vi "PlatManipbyVoltage.vi"() -> ()   [LabVIEW 2015]
uses:
  <vilib>/picture/3D Picture Control/Object/Create Object (name).vi
  <vilib>/picture/3D Picture Control/NI_3D Picture Control.lvlib
panel:
  in  "Length Y":sgl=1.0
  in  "Length X":sgl=1.0
  in  "Length Z":sgl=1.0
  in  "Tamaño de la platina":cluster{"X":sgl, "Y":sgl, "Z":sgl}={"X"=1.457233, "Y"=1.0, "Z"=1.0} {"X" scale=0.0..5.0; "Y" scale=0.0..5.0; "Z" scale=0.0..5.0}
  out "Platina":refnum<vi>(3d-picture)
  out "data":dynamicdata(graph) caption="Voltaje"
  in  "stop":bool
  # "Manipulacion de una platina virtual"
  # "Serrano Bermúdez Luis Esteban\nFecha de Entrega 13/04/2019"
  # "Descripcion:"
  # "Esta aplicacion simula una platina con un objeto 3D de una caja la cual\nse puede mover con el uso de potenciometros conectados a la tarjeta\nDAQ a partir de la medicion de voltaje a la salida de la terminal central\ndel potenciometro.\nLas gráficas del lado derecho muestra la variación del voltaje y la\ngráfica del lado derecho simula una platina que se moverá\ndependiendo del potenciometro."
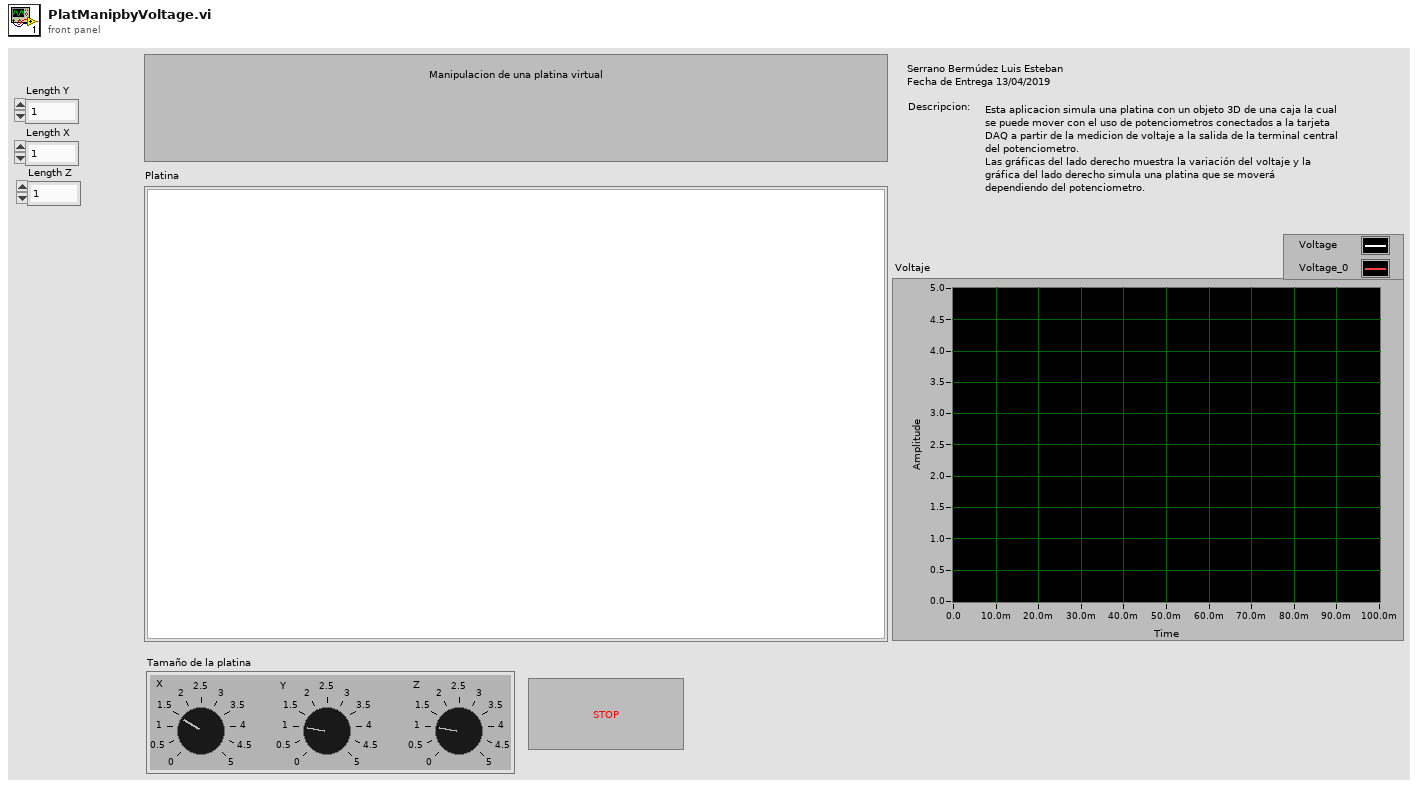
[diagram p1: front panel]
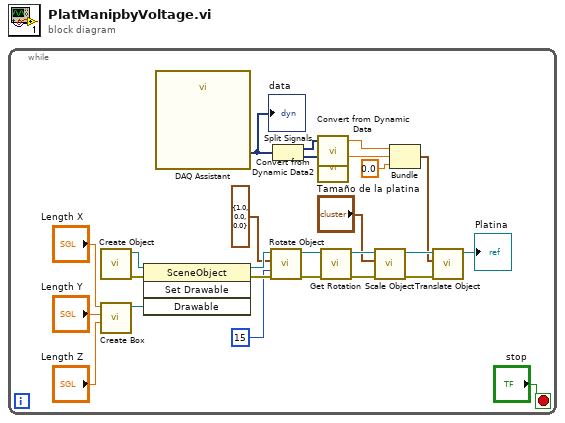
[diagram p0: block diagram]
diagram:
  n1 = while {
    stop <- "stop" stop-if-true
    n2 = call-poly <vilib>:"Create Object.vi"() -> ("error out"=w24:errorcluster, "Scene:New Object"=w25:refnum<vi>)  [unwired: 10 in]
    n3 = call <vilib>:"Create Box.vi"("Length Z"="Length Z", "Length Y"="Length Y", "Length X"="Length X") -> ("New Box Refnum"=w23:refnum<vi>)  [unwired: 7 in, 1 out]
    n4 = invoke class="SceneObject" method="Set Drawable"(reference=w25, error in=w24, "Drawable"=w23) -> (reference out=w19:refnum<vi>, error out=w18:errorcluster)  [unwired: 1 in, 2 out]
    n5 = call "DAQ Assistant"() -> ("data"=w5:dynamicdata)  [unwired: 17 in, 2 out]
    "data" <- w5
    n6 = call <vilib>:"Rotate Object.vi"("error in (no error)"=w18, "Angle"=15, "Axis"=cluster{"X":sgl, "Y":sgl, "Z":sgl} {"X"=1.0, "Y"=0.0, "Z"=0.0}, "Scene.Object In"=w19) -> ("error out"=w16:errorcluster, "Scene.Object Out"=w17:refnum<vi>)  [unwired: 6 in]
    n7 = Split Signals(w5) -> (w4:dynamicdata, w3:dynamicdata)  [unwired: 2 in]
    n8 = call "Convert from Dynamic Data"("Dynamic Data Type"=w4) -> ("Scalar"=w2:dbl)  [unwired: 3 in]
    n9 = call "Convert from Dynamic Data2"("Dynamic Data Type"=w3) -> ("Scalar"=w1:dbl)  [unwired: 3 in]
    n10 = call <vilib>:"Get Rotation.vi"("error in (no error)"=w16, "Scene Object"=w17) -> ("error out"=w14:errorcluster, "Scene Object"=w15:refnum<vi>)  [unwired: 6 in, 2 out]
    n11 = call <vilib>:"Scale Object.vi"("error in (no error)"=w14, "Scale"="Tamaño de la platina", "Scene.Object In"=w15) -> ("error out"=w11:errorcluster, "Scene.Object Out"=w12:refnum<vi>)  [unwired: 7 in]
    n12 = Bundle("Scalar"=w2, "Scalar"=w1, 0.0) -> (w6:cluster{"Scalar":dbl, "Scalar":dbl, dbl})  [unwired: 1 in]
    n13 = call <vilib>:"Translate Object.vi"("error in (no error)"=w11, "Translation"=w6, "Scene.Object In"=w12) -> ("Scene.Object Out"=→"Platina":refnum<vi>)  [unwired: 7 in, 1 out]
  }
